vi "sendMessages.vi"(8 "error in (no error)":errorcluster, 10 "messageString":string, 11 "NetworkClient in":refnum<class "NetworkServer.lvclass">) -> (0 "error out":errorcluster, 3 "NetworkClient out":refnum<class "NetworkServer.lvclass">)   [LabVIEW 2009, in "Hardware.lvlib" / "HWControllers.lvlib" / "NetworkServer.lvclass"]
uses:
  NetworkServer.lvclass
panel:
  out "time":dbl format="%.6g"
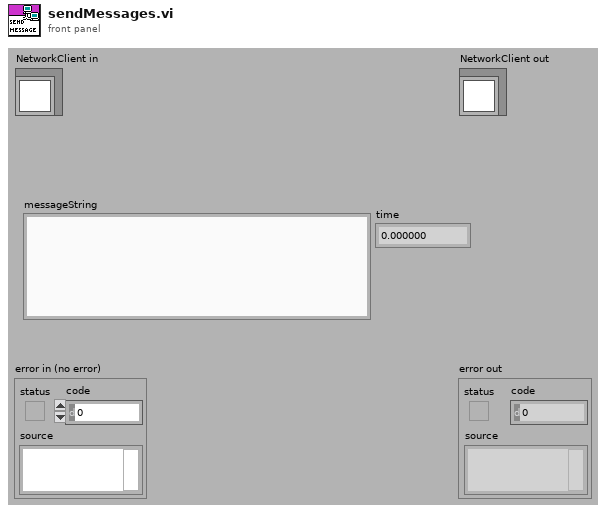
[diagram p1: front panel]
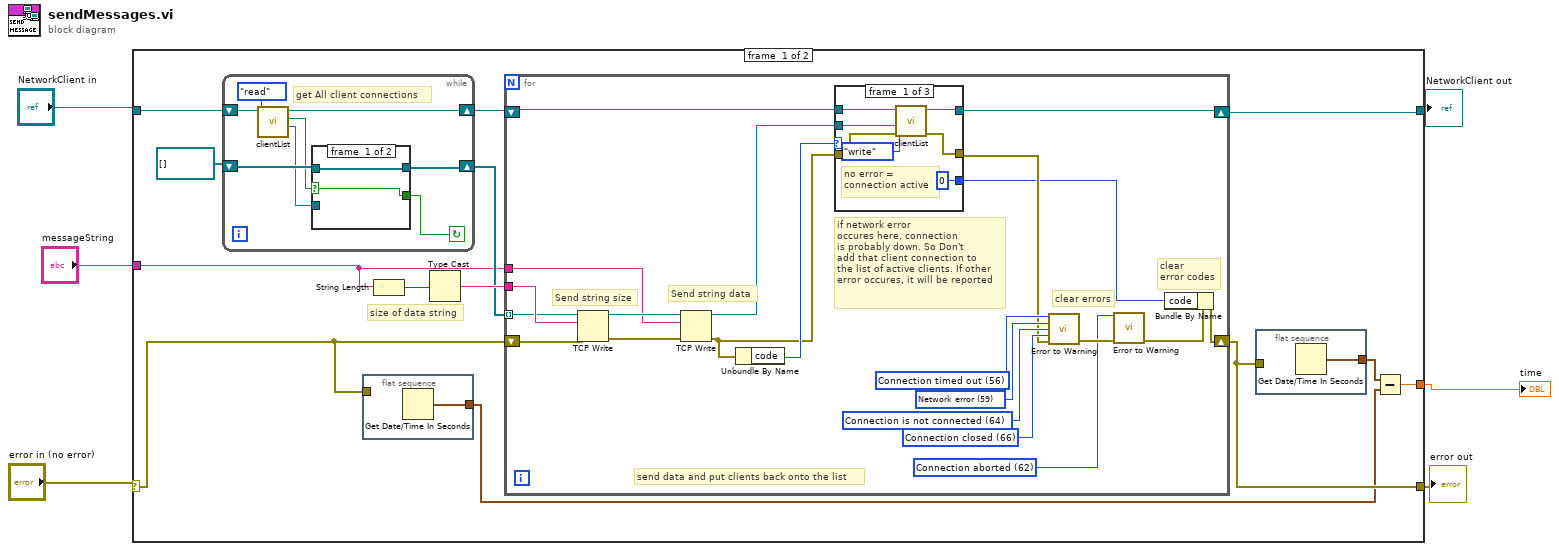
[diagram p0: block diagram]
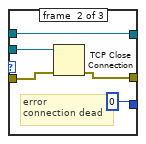
[diagram p2: hidden frame]
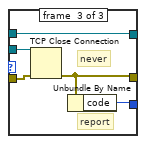
[diagram p3: hidden frame]
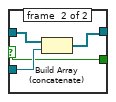
[diagram p4: hidden frame]
diagram:
  n1 = case shown="No Error" "error in (no error)" {
    selector: "error in (no error)" -> [w11 w75]
    tunnel: [w10 w75] -> w4
    tunnel: [w12 w74] -> w5
    tunnel: "NetworkClient in" -> [w14 w74]
    tunnel: "messageString" -> [w15 _]
    tunnel: [w7 _] -> w1
    frame #0 {
      # "size of data string"
      n2 = while {
        shift-right: [w65] -> w16
        shift-left: refnum<k5>[] [] ("empty") -> [w66]
        shift-right: [w61] -> w13
        shift-left: w14 -> [w64]
        stop <- w67 continue-if-true
        # "get All client connections"
        n3 = call "clientList.vi"("Enum"=enum16{"read", "write", "reset"}."read", "NetworkServer in"=w64) -> ("client"=w62:refnum<k5>, "valid?"=w63:bool, "NetworkServer out"=w61:refnum<class "NetworkServer.lvclass">)  [unwired: 6 in, 1 out]
        n4 = case shown="True" w63 {
          selector: w63 -> [w68 w71]
          tunnel: w62 -> [_ w73]
          tunnel: w66 -> [w69 w72]
          tunnel: [w68 w71] -> w67
          tunnel: [w69 w70] -> w65
          frame #0 {
          }
          frame #1 {
            n5 = Build Array (concatenate)(w72, w73) -> (w70:refnum<k5>[])
          }
        }
      }
      n6 = flat-sequence {
        tunnel: [w21] -> w8
        tunnel: w11 -> [_]
        frame #0 {
          n7 = Get Date/Time In Seconds() -> (seconds since 1Jan1904=w21:timestamp)
        }
      }
      n8 = String Length(string=w15) -> (length=w18:i32)
      n9 = Type Cast(x=w18) -> (*(type *) &x=w19:string)  [unwired: 1 in]
      n10 = for {
        tunnel: w19 -> [w40]
        tunnel: w15 -> [w39]
        tunnel: w16 -> [w38] mode=indexing
        shift-right: [w25] -> w10
        shift-left: w11 -> [w22]
        shift-right: [w37] -> w12
        shift-left: w13 -> [w36]
        w27 = 62 items=["No Error", "Argument Error", "Memory Full", "Out of Zone", "End of File", "File Already Open", "Generic File IO Error", "File Not Found", "File Permission Error", "Disk Full", "Duplicate Path", "Too Many Files Open", "Not Enabled", "Resource File Not Found", "Cannot Add Resource", "Resource Not Found", "Image Not Found", "Image Memory Error", "Pen Does Not Exist", "Config Bad Type", "Config Token Not Found", "Config Parse Error", "Config Memory Error", "Bad External Code Format", "Bad External Code Offset", "External Code Not Present", "Null Window", "Destroy Window Mixup", "Null Menu", "Print Aborted", "Bad Print Record", "Print Driver Error", "Windows Error During Print", "Memory Error During Print", "Print Dialog Error", "Generic Print Error", "Invalid Device Refnum", "Device Not Found", "Device Parameter Error", "Device Unit Error", "Can't Open Device", "Device Call Aborted", "Generic Error", "Cancelled By User", "Object ID Too Low", "Object ID Too High", "Object Not In Heap", "Unknown Heap", "Bad DefProc ID", "DefProc Not In Table", "Message Out Of Range", "Null Method", "Unknown Message", "Manager Call Not Supported", "Bad address", "Connection In progress", "Connection timed out", "Connection is already in progress", "Network attribute not supported", "Network error", "Address in use", "System out of memory", "Connection aborted", "Connection refused", "Connection is not connected", "Connection is already connected", "Connection closed", "Initialize error (interapplication manager)", "Bad occurrence", "Wait on unbound occurrence handler", "Occurrence queue overflow", "Bad path", "Semaphore not signaled", "Unrecognized type (interapplication manager)"] ("1st Error to Convert")
        w33 = 56 items=["No Error", "Argument Error", "Memory Full", "Out of Zone", "End of File", "File Already Open", "Generic File IO Error", "File Not Found", "File Permission Error", "Disk Full", "Duplicate Path", "Too Many Files Open", "Not Enabled", "Resource File Not Found", "Cannot Add Resource", "Resource Not Found", "Image Not Found", "Image Memory Error", "Pen Does Not Exist", "Config Bad Type", "Config Token Not Found", "Config Parse Error", "Config Memory Error", "Bad External Code Format", "Bad External Code Offset", "External Code Not Present", "Null Window", "Destroy Window Mixup", "Null Menu", "Print Aborted", "Bad Print Record", "Print Driver Error", "Windows Error During Print", "Memory Error During Print", "Print Dialog Error", "Generic Print Error", "Invalid Device Refnum", "Device Not Found", "Device Parameter Error", "Device Unit Error", "Can't Open Device", "Device Call Aborted", "Generic Error", "Cancelled By User", "Object ID Too Low", "Object ID Too High", "Object Not In Heap", "Unknown Heap", "Bad DefProc ID", "DefProc Not In Table", "Message Out Of Range", "Null Method", "Unknown Message", "Manager Call Not Supported", "Bad address", "Connection In progress", "Connection timed out", "Connection is already in progress", "Network attribute not supported", "Network error", "Address in use", "System out of memory", "Connection aborted", "Connection refused", "Connection is not connected", "Connection is already connected", "Connection closed", "Initialize error (interapplication manager)", "Bad occurrence", "Wait on unbound occurrence handler", "Occurrence queue overflow", "Bad path", "Semaphore not signaled", "Unrecognized type (interapplication manager)"] ("1st Error to Convert")
        w32 = 59 items=["No Error", "Argument Error", "Memory Full", "Out of Zone", "End of File", "File Already Open", "Generic File IO Error", "File Not Found", "File Permission Error", "Disk Full", "Duplicate Path", "Too Many Files Open", "Not Enabled", "Resource File Not Found", "Cannot Add Resource", "Resource Not Found", "Image Not Found", "Image Memory Error", "Pen Does Not Exist", "Config Bad Type", "Config Token Not Found", "Config Parse Error", "Config Memory Error", "Bad External Code Format", "Bad External Code Offset", "External Code Not Present", "Null Window", "Destroy Window Mixup", "Null Menu", "Print Aborted", "Bad Print Record", "Print Driver Error", "Windows Error During Print", "Memory Error During Print", "Print Dialog Error", "Generic Print Error", "Invalid Device Refnum", "Device Not Found", "Device Parameter Error", "Device Unit Error", "Can't Open Device", "Device Call Aborted", "Generic Error", "Cancelled By User", "Object ID Too Low", "Object ID Too High", "Object Not In Heap", "Unknown Heap", "Bad DefProc ID", "DefProc Not In Table", "Message Out Of Range", "Null Method", "Unknown Message", "Manager Call Not Supported", "Bad address", "Connection In progress", "Connection timed out", "Connection is already in progress", "Network attribute not supported", "Network error", "Address in use", "System out of memory", "Connection aborted", "Connection refused", "Connection is not connected", "Connection is already connected", "Connection closed", "Initialize error (interapplication manager)", "Bad occurrence", "Wait on unbound occurrence handler", "Occurrence queue overflow", "Bad path", "Semaphore not signaled", "Unrecognized type (interapplication manager)"] ("1st Error to Convert")
        w30 = 66 items=["No Error", "Argument Error", "Memory Full", "Out of Zone", "End of File", "File Already Open", "Generic File IO Error", "File Not Found", "File Permission Error", "Disk Full", "Duplicate Path", "Too Many Files Open", "Not Enabled", "Resource File Not Found", "Cannot Add Resource", "Resource Not Found", "Image Not Found", "Image Memory Error", "Pen Does Not Exist", "Config Bad Type", "Config Token Not Found", "Config Parse Error", "Config Memory Error", "Bad External Code Format", "Bad External Code Offset", "External Code Not Present", "Null Window", "Destroy Window Mixup", "Null Menu", "Print Aborted", "Bad Print Record", "Print Driver Error", "Windows Error During Print", "Memory Error During Print", "Print Dialog Error", "Generic Print Error", "Invalid Device Refnum", "Device Not Found", "Device Parameter Error", "Device Unit Error", "Can't Open Device", "Device Call Aborted", "Generic Error", "Cancelled By User", "Object ID Too Low", "Object ID Too High", "Object Not In Heap", "Unknown Heap", "Bad DefProc ID", "DefProc Not In Table", "Message Out Of Range", "Null Method", "Unknown Message", "Manager Call Not Supported", "Bad address", "Connection In progress", "Connection timed out", "Connection is already in progress", "Network attribute not supported", "Network error", "Address in use", "System out of memory", "Connection aborted", "Connection refused", "Connection is not connected", "Connection is already connected", "Connection closed", "Initialize error (interapplication manager)", "Bad occurrence", "Wait on unbound occurrence handler", "Occurrence queue overflow", "Bad path", "Semaphore not signaled", "Unrecognized type (interapplication manager)"] ("2nd Error to Convert")
        w31 = 64 items=["No Error", "Argument Error", "Memory Full", "Out of Zone", "End of File", "File Already Open", "Generic File IO Error", "File Not Found", "File Permission Error", "Disk Full", "Duplicate Path", "Too Many Files Open", "Not Enabled", "Resource File Not Found", "Cannot Add Resource", "Resource Not Found", "Image Not Found", "Image Memory Error", "Pen Does Not Exist", "Config Bad Type", "Config Token Not Found", "Config Parse Error", "Config Memory Error", "Bad External Code Format", "Bad External Code Offset", "External Code Not Present", "Null Window", "Destroy Window Mixup", "Null Menu", "Print Aborted", "Bad Print Record", "Print Driver Error", "Windows Error During Print", "Memory Error During Print", "Print Dialog Error", "Generic Print Error", "Invalid Device Refnum", "Device Not Found", "Device Parameter Error", "Device Unit Error", "Can't Open Device", "Device Call Aborted", "Generic Error", "Cancelled By User", "Object ID Too Low", "Object ID Too High", "Object Not In Heap", "Unknown Heap", "Bad DefProc ID", "DefProc Not In Table", "Message Out Of Range", "Null Method", "Unknown Message", "Manager Call Not Supported", "Bad address", "Connection In progress", "Connection timed out", "Connection is already in progress", "Network attribute not supported", "Network error", "Address in use", "System out of memory", "Connection aborted", "Connection refused", "Connection is not connected", "Connection is already connected", "Connection closed", "Initialize error (interapplication manager)", "Bad occurrence", "Wait on unbound occurrence handler", "Occurrence queue overflow", "Bad path", "Semaphore not signaled", "Unrecognized type (interapplication manager)"] ("1st Error to Convert")
        # "clear\nerror codes"
        # "clear errors"
        # "if network error \noccures here, connection\nis probably down. So Don't\nadd that client connection to\nthe list of active clients. If other\nerror occures, it will be reported"
        # "send data and put clients back onto the list"
        # "Send string data"
        # "Send string size"
        n11 = TCP Write(connection ID=w38, data in=w40, error in (no error)=w22) -> (connection ID out=w41:refnum<k5>, error out=w42:errorcluster)  [unwired: 1 in, 1 out]
        n12 = TCP Write(connection ID=w41, data in=w39, error in (no error)=w42) -> (connection ID out=w35:refnum<k5>, error out=w23:errorcluster)  [unwired: 1 in, 1 out]
        n13 = Unbundle By Name(w23) -> ("code"=w34:i32)
        n14 = case shown="56, 59, 62, 64, 66" w34 {
          tunnel: [w49 w54 w57] -> w37
          tunnel: w36 -> [w48 w54 w57]
          tunnel: w35 -> [w47 w53 w59]
          tunnel: w23 -> [w46 w52 w58]
          tunnel: [w45 w51 w56] -> w29
          tunnel: [0 0 w55] -> w24
          frame #0 {
            # "no error = \nconnection active"
            n15 = call "clientList.vi"("error in (no error)"=w46, "new client"=w47, "Enum"=enum16{"read", "write", "reset"}."write", "NetworkServer in"=w48) -> ("error out"=w45:errorcluster, "NetworkServer out"=w49:refnum<class "NetworkServer.lvclass">)  [unwired: 4 in, 2 out]
          }
          frame #1 {
            # "error\nconnection dead"
            n16 = TCP Close Connection(connection ID=w53, error in (no error)=w52) -> (error out=w51:errorcluster)  [unwired: 1 in, 1 out]
          }
          frame #2 {
            # "never"
            # "report"
            n17 = TCP Close Connection(connection ID=w59, error in (no error)=w58) -> (error out=w56:errorcluster)  [unwired: 1 in, 1 out]
            n18 = Unbundle By Name(w56) -> ("code"=w55:i32)
          }
        }
        n19 = call <vilib>:"Error to Warning.vi"("1st Error to Convert"=w33, "2nd Error to Convert"=w32, "3rd Error to Convert"=w31, "4th Error to Convert"=w30, "error in"=w29) -> ("warning out"=w28:errorcluster)  [unwired: 10 out]
        n20 = call <vilib>:"Error to Warning.vi"("1st Error to Convert"=w27, "error in"=w28) -> ("warning out"=w26:errorcluster)  [unwired: 3 in, 10 out]
        n21 = Bundle By Name(cluster=w26, "code"=w24) -> (w25:errorcluster)
      }
      n22 = flat-sequence {
        tunnel: [w20] -> w9
        tunnel: w10 -> [_]
        frame #0 {
          n23 = Get Date/Time In Seconds() -> (seconds since 1Jan1904=w20:timestamp)
        }
      }
      n24 = Subtract(x=w9, y=w8) -> (x-y=w7:dbl)
    }
    frame #1 {
    }
  }
  "error out" <- w4
  "NetworkClient out" <- w5
  "time" <- w1
